vi "TriggerSpectraWizInit.vi"(8 "error in (no error)":errorcluster, 11 "Microscope in":refnum<class "Microscope.lvclass">) -> (0 "error out":errorcluster, 3 "Microscope out":refnum<class "Microscope.lvclass">)   [LabVIEW 2012, in "Microscope.lvclass"]
uses:
  classes/Microscope.lvclass
  classes/Microscope.lvclass/Microscope.ctl
  Spectrometer/Events/SpectrometerEvents.ctl
  Spectrometer/SpectrometerSpectraWiz.llb/StellarNet Globals.vi
  variables/GlobalUI.vi
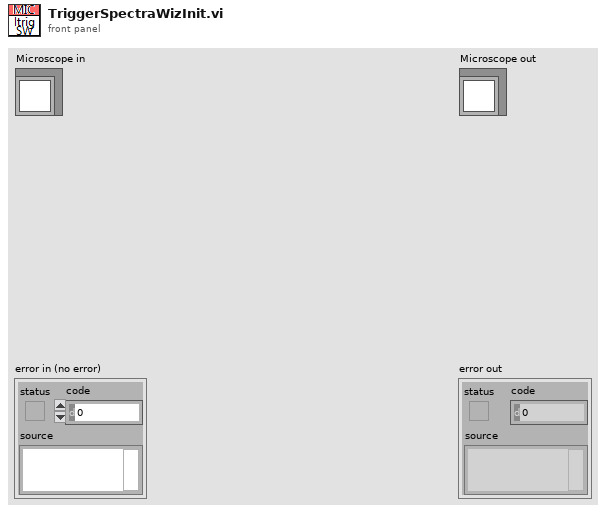
[diagram p1: front panel]
types:
  T1 = typedef "SpectrometerEvents.ctl" = enum16{"TimeOut", "Init Programmatically", "Init Button", "Init Background", "Acquire Background", "Acquire"}
  T2 = typedef "DetectorType.ctl" = enum16{"PMT", "SpectraWiz"}
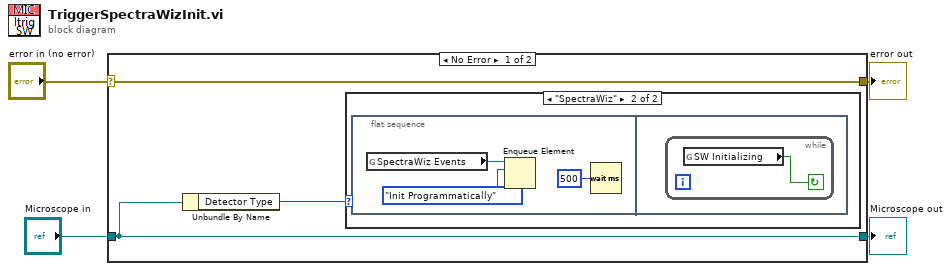
[diagram p0: block diagram]
diagram:
  n1 = case shown="No Error" "error in (no error)" {
    selector: "error in (no error)" -> [w7 w13]
    tunnel: [w7 w13] -> w3
    tunnel: [w6 w12] -> w1
    tunnel: "Microscope in" -> [w6 w12]
    frame No Error {
      n2 = Unbundle By Name(w6) -> ("Detector Type"=w5:T2)
      n3 = case shown="\"SpectraWiz\"" w5 {
        frame "PMT", Default {
        }
        frame "SpectraWiz" {
          n4 = flat-sequence {
            frame #0 {
              n5 = global read "StellarNet Globals.vi" "SpectraWiz Events"() -> (w10:refnum<queue>)
              n6 = Enqueue Element(queue=w10, element=SpectrometerEvents."Init Programmatically") -> ()  [unwired: 2 in, 3 out]
              n7 = Wait (ms)(milliseconds to wait=u32 500) -> ()  [unwired: 1 out]
            }
            frame #1 {
              n8 = while {
                stop <- w11 continue-if-true
                n9 = global read "GlobalUI.vi" "SW Initializing"() -> (w11:bool)
              }
            }
          }
        }
      }
    }
    frame Error {
    }
  }
  "error out" <- w3
  "Microscope out" <- w1
